vi "Inst_DS360.vi"(8 "error in":errorcluster, 10 "All Message Queues in":T1, 11 "Prueba05 in":refnum<class "Prueba05.lvclass">) -> (0 "error out":errorcluster)   [LabVIEW 2019, in "Prueba05.lvclass"]
uses:
  Prueba05.lvclass
  QMH/Message Queue/All Message Queues.ctl
  QMH/Message Queue/Message Cluster.ctl
  Prueba05.lvclass/Prueba05.ctl
  ClusterGEN.ctl
  <vilib>/Utility/error.llb/Error Cluster From Error Code.vi
  QMH/Message Queue/Enqueue Message (Single).vi
  <vilib>/ErrorRing/Error Ring.xnode
  QMH/Message Queue/Message Queue.lvlib
  Instrumento/DS360/DS360.lvclass
panel:
  out "All States":string[](array[string])
  out "Actual State":string
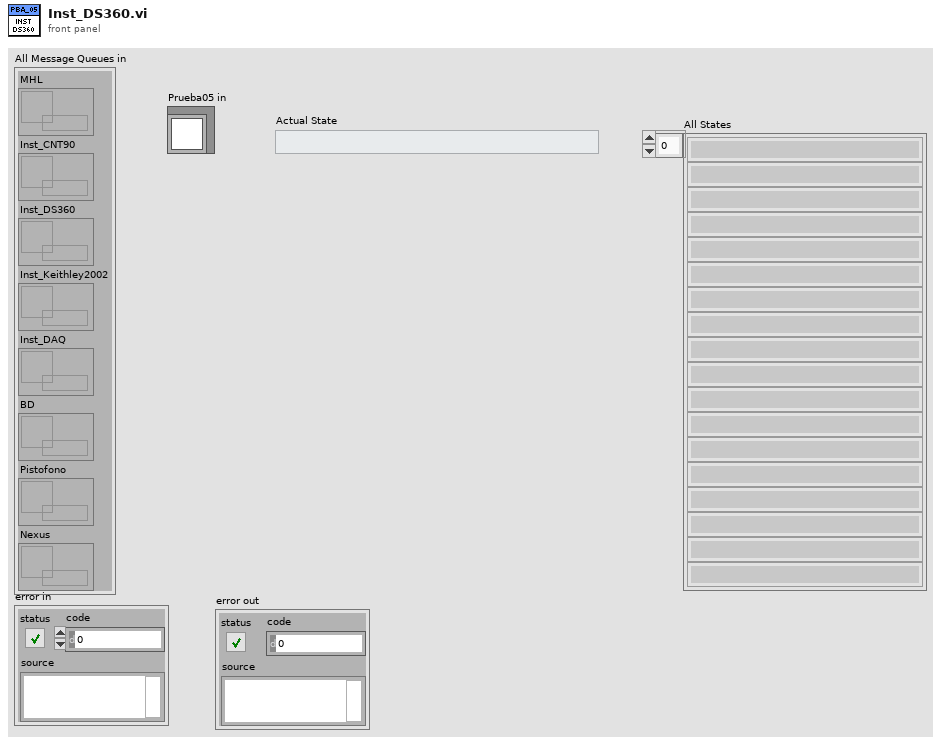
[diagram p1: front panel]
types:
  T1 = typedef "Message Queue.lvlib/All Message Queues.ctl" = cluster{"MHL":refnum<queue>, "Inst_CNT90":refnum<queue>, "Inst_DS360":refnum<queue>, "Inst_Keithley2002":refnum<queue>, "Inst_DAQ":refnum<queue>, "BD":refnum<queue>, "Pistofono":refnum<queue>, "Nexus":refnum<queue>}
  T2 = typedef "Prueba05.lvclass/ClusterGEN.ctl" = cluster{"frec":dbl, "amp":dbl}
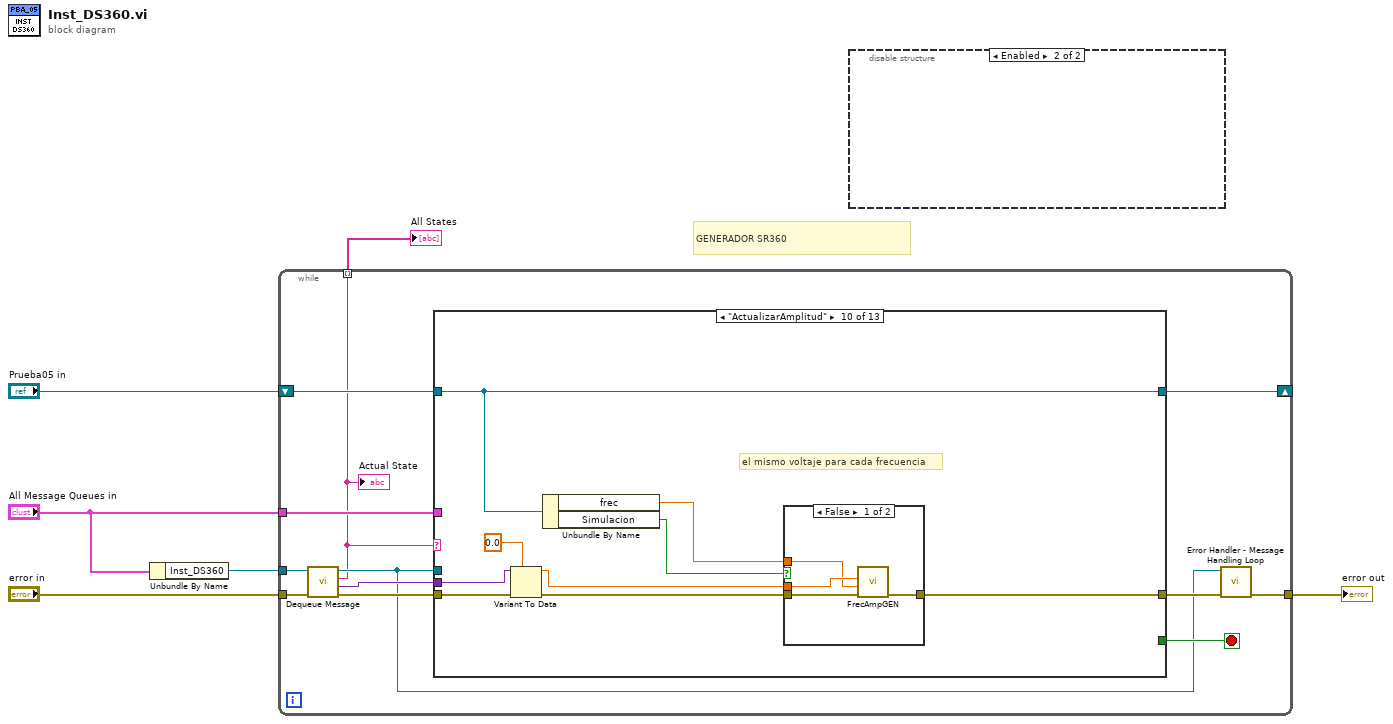
[diagram p0: block diagram]
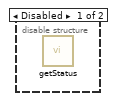
[diagram p2: hidden frame]
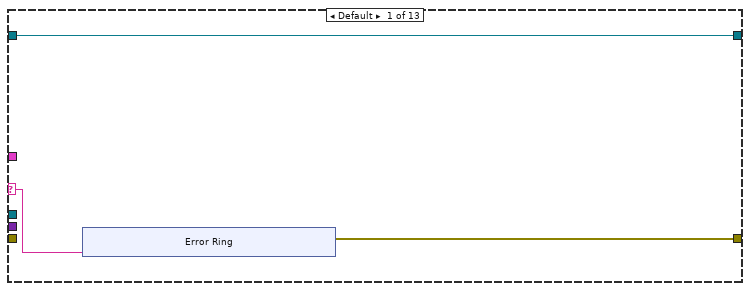
[diagram p3: hidden frame]
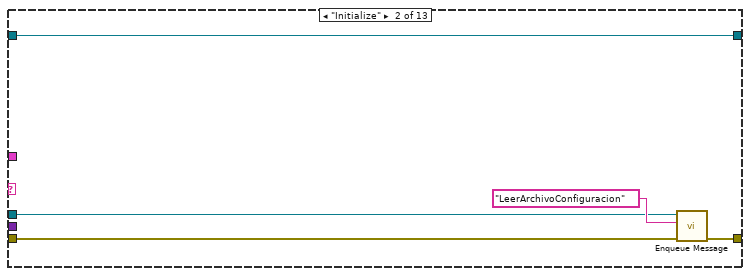
[diagram p4: hidden frame]
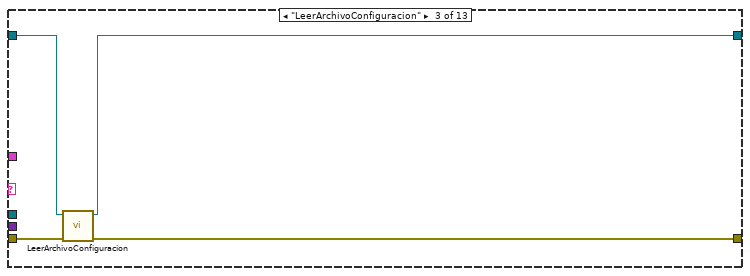
[diagram p5: hidden frame]
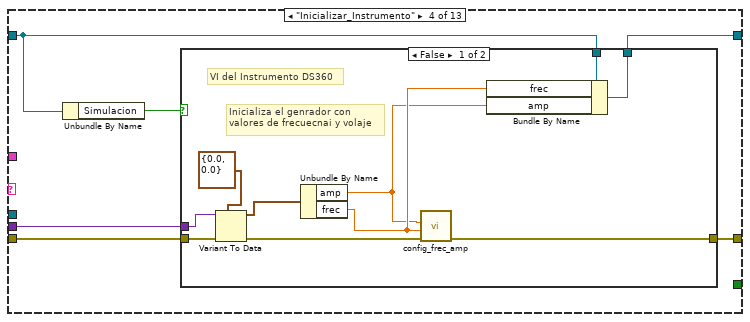
[diagram p6: hidden frame]
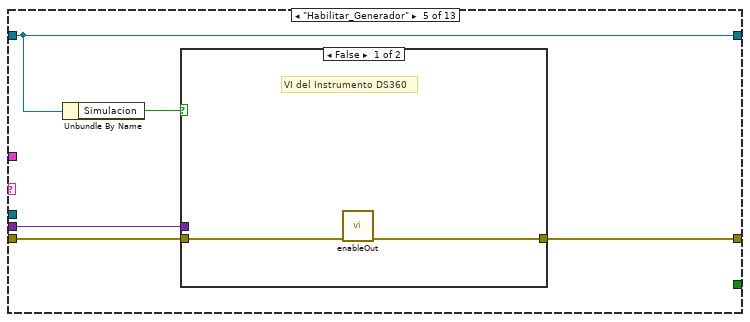
[diagram p8: hidden frame]
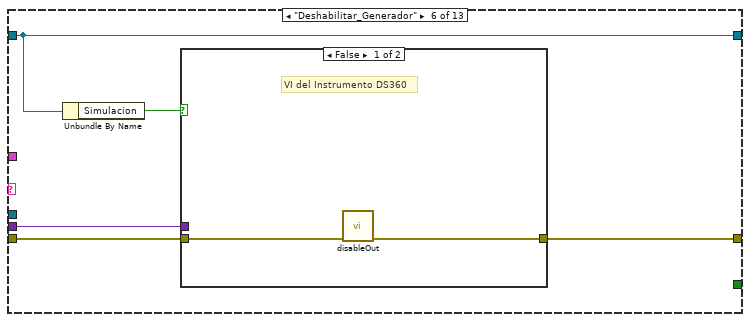
[diagram p10: hidden frame]
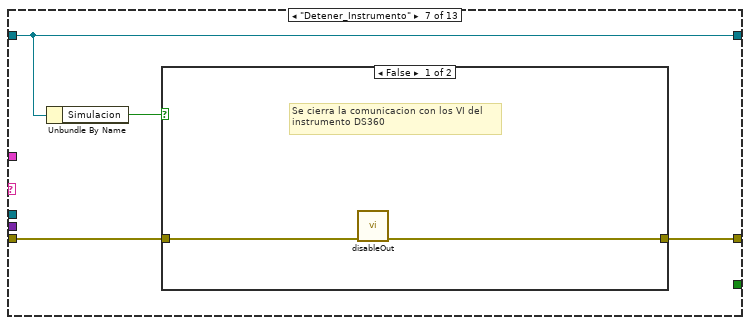
[diagram p12: hidden frame]
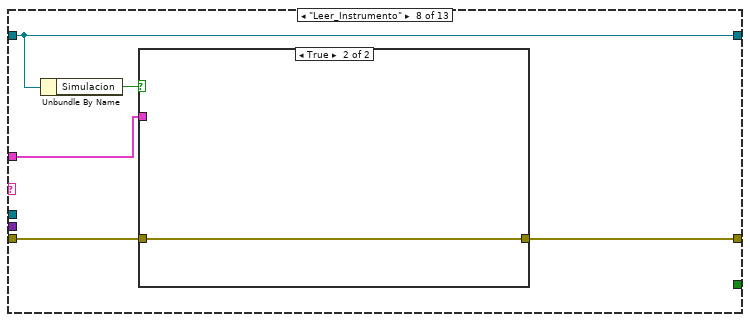
[diagram p14: hidden frame]
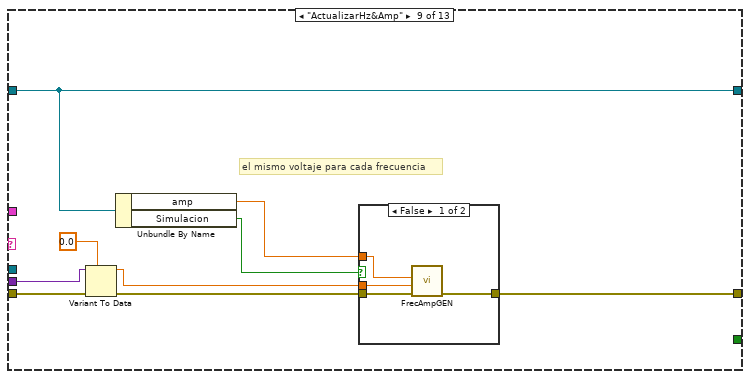
[diagram p16: hidden frame]
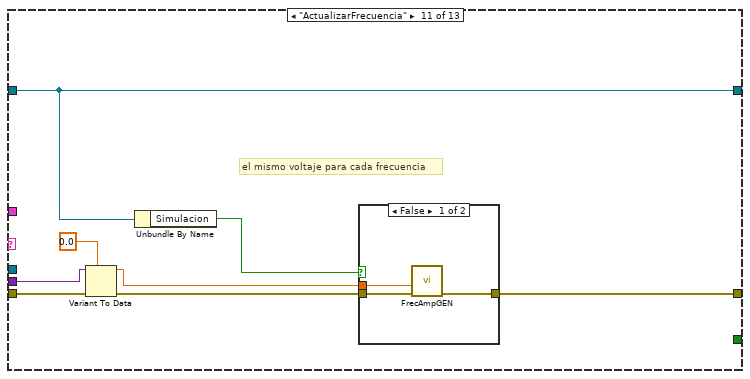
[diagram p19: hidden frame]
diagram:
  # "GENERADOR SR360"
  n1 = Unbundle By Name("All Message Queues in") -> ("Inst_DS360"=w4:refnum<queue>)
  n2 = while {
    tunnel: "error in" -> [w18]
    tunnel: w4 -> [w17]
    tunnel: "All Message Queues in" -> [w16]
    tunnel: [w9] -> w2
    shift-right: [w12] -> _
    shift-left: "Prueba05 in" -> [w15]
    tunnel: [w7] -> w1 mode=indexing
    stop <- w11 stop-if-true
    n3 = call "Dequeue Message.vi"("error in (no error)"=w18, "Message Queue"=w17) -> ("error out"=w13:errorcluster, "Message Data"=w14:variant, "Message"=w7:string, "dup Message Queue"=w8:refnum<queue>)  [unwired: 6 in]
    "Actual State" <- w7
    n4 = case shown="\"ActualizarAmplitud\"" w7 {
      selector: w7 -> [w21 _ _ _ _ _ _ _ _ _ _ w128 _]
      tunnel: w16 -> [_ _ _ _ _ _ _ w82 _ _ _ w127 _]
      tunnel: w15 -> [w19 w33 w34 w39 w58 w66 w74 w81 w90 w104 w117 w135 w137]
      tunnel: w8 -> [_ w29 _ _ _ _ _ _ _ _ _ _ w139]
      tunnel: w14 -> [_ _ _ w41 w57 w65 _ _ w91 w105 w118 w132 _]
      tunnel: w13 -> [_ w30 w36 w40 w56 w64 w72 w83 w92 w106 w119 w133 w140]
      tunnel: [w20 w31 w37 w43 w60 w68 w75 w79 w94 w108 w121 w130 w136] -> w10
      tunnel: [w19 w33 w35 w38 w58 w66 w74 w81 w90 w104 w117 w135 w137] -> w12
      tunnel: [_ _ _ _ _ _ _ _ _ _ _ _ TRUE] -> w11
      frame Default {
        n5 = xnode "Error Ring"("parameter 0"=w21) -> ("error out"=w20:errorcluster)
      }
      frame "Initialize" {
        n6 = call-poly "Enqueue Message.vi"("error in (no error)"=w30, "Message"="LeerArchivoConfiguracion", "Message Queue"=w29) -> ("error out"=w31:errorcluster)  [unwired: 7 in, 1 out]
      }
      frame "LeerArchivoConfiguracion" {
        n7 = call "LeerArchivoConfiguracion.vi"("error in"=w36, "Prueba05 in"=w34) -> ("error out"=w37:errorcluster, "Prueba05 out"=w35:refnum<class "Prueba05.lvclass">)  [unwired: 8 in]
      }
      frame "Inicializar_Instrumento" {
        n8 = Unbundle By Name(w39) -> ("Simulacion"=w42:bool)
        n9 = case shown="False" w42 {
          tunnel: [w52 w55] -> w43
          tunnel: w40 -> [w53 w55]
          tunnel: w41 -> [w50 _]
          tunnel: w39 -> [w47 w54]
          tunnel: [w46 w54] -> w38
          frame False {
            # "Inicializa el genrador con \nvalores de frecuecnai y volaje"
            # "VI del Instrumento DS360"
            n10 = Variant To Data(error in=w53, type=T2 {"frec"=0.0, "amp"=0.0} ("clusterGEN"), Variant=w50) -> (data=w49:T2, error out=w51:errorcluster)
            n11 = Unbundle By Name(w49) -> ("amp"=w44:dbl, "frec"=w45:dbl)
            n12 = call "config_frec_amp.vi"("error in (no error)"=w51, "Frec (Hz)"=w45, "Amplitud (Vrms)"=w44) -> ("error out"=w52:errorcluster)  [unwired: 7 in, 1 out]
            n13 = Bundle By Name(cluster=w47, "frec"=w45, "amp"=w44) -> (w46:refnum<class "Prueba05.lvclass">)
          }
          frame True {
            # "Simulacion"
          }
        }
      }
      frame "Habilitar_Generador" {
        n14 = Unbundle By Name(w58) -> ("Simulacion"=w59:bool)
        n15 = case shown="False" w59 {
          tunnel: [w61 w63] -> w60
          tunnel: w56 -> [w62 w63]
          tunnel: w57 -> [_ _]
          frame False {
            # "VI del Instrumento DS360"
            n16 = call "enableOut.vi"("error in (no error)"=w62) -> ("error out"=w61:errorcluster)  [unwired: 9 in, 1 out]
          }
          frame True {
            # "Simulacion"
          }
        }
      }
      frame "Deshabilitar_Generador" {
        n17 = Unbundle By Name(w66) -> ("Simulacion"=w67:bool)
        n18 = case shown="False" w67 {
          tunnel: [w69 w71] -> w68
          tunnel: w64 -> [w70 w71]
          tunnel: w65 -> [_ _]
          frame False {
            # "VI del Instrumento DS360"
            n19 = call "disableOut.vi"("error in (no error)"=w70) -> ("error out"=w69:errorcluster)  [unwired: 9 in, 1 out]
          }
          frame True {
            # "Simulacion"
          }
        }
      }
      frame "Detener_Instrumento" {
        n20 = Unbundle By Name(w74) -> ("Simulacion"=w73:bool)
        n21 = case shown="False" w73 {
          tunnel: [w77 w78] -> w75
          tunnel: w72 -> [w76 w78]
          frame False {
            # "Se cierra la comunicacion con los VI del\ninstrumento DS360"
            n22 = call "disableOut.vi"("error in (no error)"=w76) -> ("error out"=w77:errorcluster)  [unwired: 9 in, 1 out]
          }
          frame True {
            # "Simulacion"
          }
        }
      }
      frame "Leer_Instrumento" {
        n23 = Unbundle By Name(w81) -> ("Simulacion"=w80:bool)
        n24 = case shown="True" w80 {
          tunnel: [w84 w85] -> w79
          tunnel: w83 -> [w84 w85]
          tunnel: w82 -> [_ _]
          frame False {
          }
          frame True {
          }
        }
      }
      frame "ActualizarHz&Amp" {
        # "el mismo voltaje para cada frecuencia"
        n25 = Variant To Data(error in=w92, type=0.0, Variant=w91) -> (data=w87:dbl, error out=w93:errorcluster)
        n26 = Unbundle By Name(w90) -> ("amp"=w89:dbl, "Simulacion"=w86:bool)
        n27 = case shown="False" w86 {
          tunnel: [w98 w99] -> w94
          tunnel: w93 -> [w97 w99]
          tunnel: w89 -> [w96 _]
          tunnel: w87 -> [w95 _]
          frame False {
            n28 = call "FrecAmpGEN.vi"("error in (no error)"=w97, "Frec (Hz)"=w95, "Amplitud (Vrms)"=w96) -> ("error out"=w98:errorcluster)  [unwired: 7 in, 1 out]
          }
          frame True {
            # "Simlacion"
          }
        }
      }
      frame "ActualizarAmplitud" {
        # "el mismo voltaje para cada frecuencia"
        n29 = Variant To Data(error in=w106, type=0.0, Variant=w105) -> (data=w102:dbl, error out=w107:errorcluster)
        n30 = Unbundle By Name(w104) -> ("frec"=w100:dbl, "Simulacion"=w101:bool)
        n31 = case shown="False" w101 {
          tunnel: [w112 w113] -> w108
          tunnel: w107 -> [w111 w113]
          tunnel: w102 -> [w110 _]
          tunnel: w100 -> [w109 _]
          frame False {
            n32 = call "FrecAmpGEN.vi"("error in (no error)"=w111, "Frec (Hz)"=w109, "Amplitud (Vrms)"=w110) -> ("error out"=w112:errorcluster)  [unwired: 7 in, 1 out]
          }
          frame True {
            # "Simlacion"
          }
        }
      }
      frame "ActualizarFrecuencia" {
        # "el mismo voltaje para cada frecuencia"
        n33 = Variant To Data(error in=w119, type=0.0, Variant=w118) -> (data=w115:dbl, error out=w120:errorcluster)
        n34 = Unbundle By Name(w117) -> ("Simulacion"=w114:bool)
        n35 = case shown="False" w114 {
          tunnel: [w124 w125] -> w121
          tunnel: w120 -> [w123 w125]
          tunnel: w115 -> [w122 _]
          frame False {
            n36 = call "FrecAmpGEN.vi"("error in (no error)"=w123, "Frec (Hz)"=w122) -> ("error out"=w124:errorcluster)  [unwired: 8 in, 1 out]
          }
          frame True {
            # "Simlacion"
          }
        }
      }
      frame "Error" {
        n37 = Unbundle By Name(w127) -> ("MHL"=w126:refnum<queue>)
        n38 = Variant To Data(error in=w133, type=errorcluster {"status"=FALSE, "code"=0, "source"=""} ("error constant"), Variant=w132) -> (data=w129:errorcluster, error out=w131:errorcluster)
        n39 = call-poly "Enqueue Message.vi"("error in (no error)"=w131, "Message Data"=w129, "Message"=w128, "Message Queue"=w126) -> ("error out"=w130:errorcluster)  [unwired: 6 in, 1 out]
      }
      frame "Exit" {
        n40 = Release Queue(queue=w139, error in (no error)=w140) -> (error out=w136:errorcluster)  [unwired: 1 in, 2 out]
      }
    }
    n41 = call "Error Handler - Message Handling Loop.vi"("error in (no error)"=w10, "Message Queue"=w8) -> ("dup error in"=w9:errorcluster)  [unwired: 8 in, 1 out]
  }
  "error out" <- w2
  "All States" <- w1
  n42 = disable-structure shown="Enabled" {
    frame Disabled {
      n43 = call "getStatus.vi"() -> ()  [unwired: 9 in, 3 out]
    }
    frame Enabled {
    }
  }
